vi "Get Default Type and Value.vi"(7 "Test Executive Builder Data Type Handler in":refnum<class "Test Executive Builder Data Type Handler.lvclass">) -> (2 "Default Value":variant, 3 "Default Type":string="Floating Point")   [LabVIEW 2017, in "Test Executive Builder Data Type Handler.lvclass"]
uses:
  <vilib>/gpm_packages/@cs/Test-executive-builder/Source/Data Type Handler/Test Executive Builder Data Type Handler.lvclass
  <vilib>/gpm_packages/@cs/Test-executive-builder/Source/Test Executive Builder Dialogs/Float Type View/Float Type View.lvclass
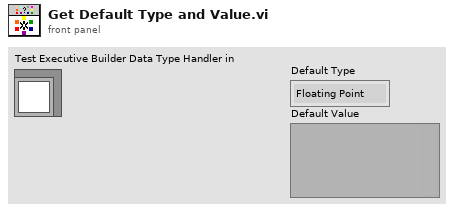
[diagram p1: front panel]
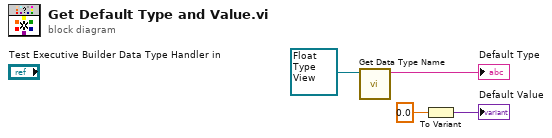
[diagram p0: block diagram]
diagram:
  n1 = call-dynamic "Get Data Type Name.vi"("String Type View in"=refnum<class "Float Type View.lvclass"> refnum ("Float Type View.lvclass")) -> ("Data Type Name"=→"Default Type":string)  [unwired: 10 in]
  n2 = To Variant(anything=0.0) -> (Variant=→"Default Value":variant)
